vi "DAQNavi Create Channel(AO-Current).vi"(0 "task in":i32=-1, 5 "physical channels":string="DemoDevice,BID#0/ao0", 7 "value range":string(combo)="Omit", 11 "error in (no error)":errorcluster) -> (4 "task out":i32, 15 "error out":errorcluster)   [LabVIEW 2020]
uses:
  DAQNavi_LV.dll
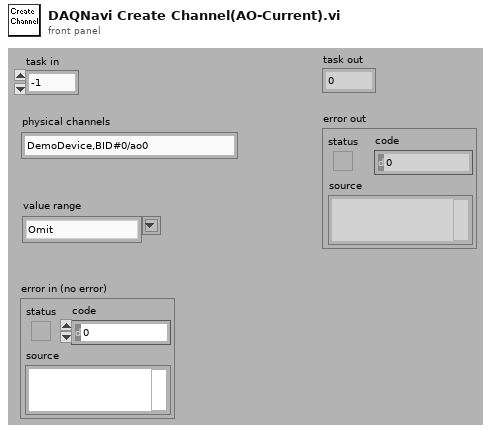
[diagram p1: front panel]
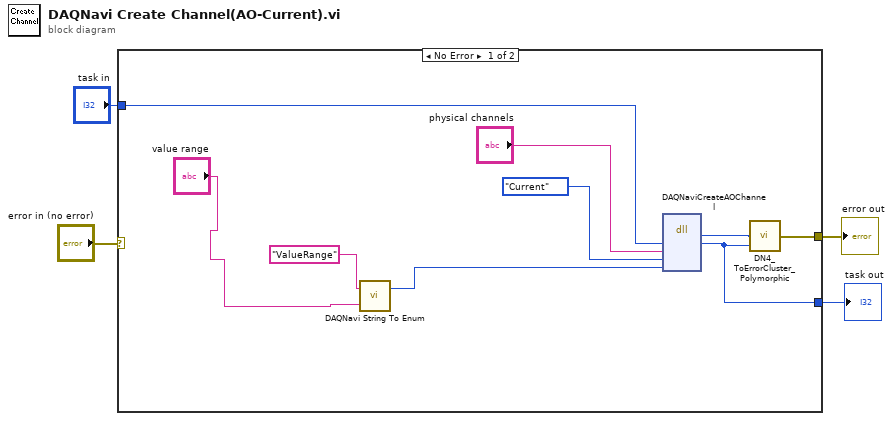
[diagram p0: block diagram]
diagram:
  n1 = case shown="No Error" "error in (no error)" {
    selector: "error in (no error)" -> [_ w14]
    tunnel: "task in" -> [w13 w15]
    tunnel: [w9 w14] -> w2
    tunnel: [w8 w15] -> w1
    frame No Error {
      n2 = call "DAQNavi String To Enum.vi"("enumString"="value range", "enumTypeName"="ValueRange") -> ("enumValue"=w6:i32)  [unwired: 1 out]
      n3 = dll-call lib="DAQNavi_LV.dll" fn="DAQNaviCreateAOChannel"("taskID"=w13, "physicalChannel"="physical channels", "type"=enum32{"Voltage", "Temperature", "Current"}."Current", "valueRange"=w6) -> ("return type"=w10:i32, "taskID"=w8:i32)  [unwired: 5 in, 3 out]
      n4 = call "DN4_ToErrorCluster_Polymorphic.vi"("task id"=w8, "error code"=w10) -> ("error out"=w9:errorcluster)  [unwired: 3 out]
    }
    frame Error {
    }
  }
  "error out" <- w2
  "task out" <- w1
